vi "load_data.vi"(0 "datasource_pdf in":refnum<class "datasource_pdf.lvclass">, 11 "error in (no error)":errorcluster) -> (4 "datasource_pdf out":refnum<class "datasource_pdf.lvclass">, 6 "document":refnum<class "data_document.lvclass">[](array[class]), 15 "error out":errorcluster)   [LabVIEW 2020, in "datasource_pdf.lvclass"]
uses:
  datasource_pdf.lvclass
  data/data_document/data_document.lvclass
  datasource_pdf.lvclass/datasource_pdf.ctl
  models/message_image/message_image.lvclass
  D:/Personal/LabVIEW LLMs/src/models/abstract_message_base/abstract_message_base.lvclass
  models/message_image/create_image_message.vi
  models/message_text/get_text_message_value.vi
  utilities/pdf_utility/pdf_utility.lvlib
  models/abstract_llm_chatcompletion/abstract_llm_chatcompletion.lvclass
  models/message_text/message_text.lvclass
panel:
  out "pdf_path":string="  "
  # "Reading context from PDF using LLM"
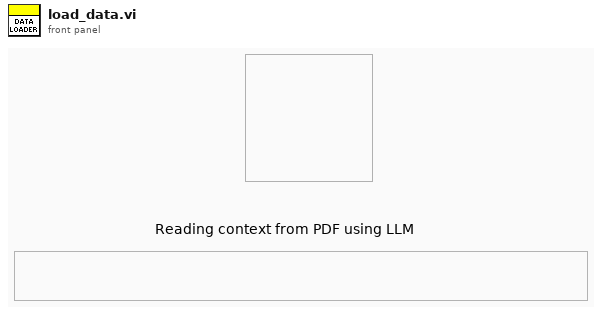
[diagram p1: front panel]
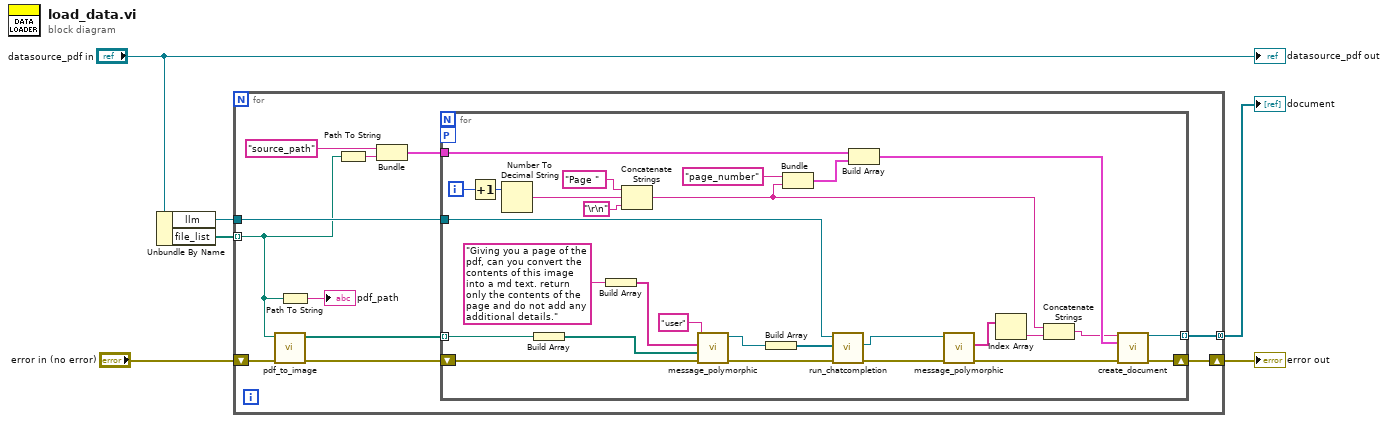
[diagram p0: block diagram]
diagram:
  n1 = Unbundle By Name("datasource_pdf in") -> ("llm"=w2:refnum<class "abstract_llm_base.lvclass">, "file_list"=w3:path[])
  n2 = for {
    shift-right: [w16] -> w4
    shift-left: "error in (no error)" -> [w17]
    tunnel: w3 -> [w7] mode=indexing
    tunnel: w2 -> [w12]
    tunnel: [w9] -> w1 mode=concatenating
    n3 = call "pdf_to_image.vi"("error in (no error)"=w17, "PDF File Path"=w7) -> ("error out"=w13:errorcluster, "Generated Images"=w11:path[])  [unwired: 8 in]
    n4 = Path To String(path=w7) -> (string=→"pdf_path":string)
    n5 = Path To String(path=w7) -> (string=w14:string)
    n6 = Bundle("source_path", w14) -> (w10:cluster{string, string})  [unwired: 1 in]
    n7 = for {
      tunnel: w12 -> [w42]
      shift-right: [w45] -> w16
      shift-left: w13 -> [w44]
      tunnel: w11 -> [w38] mode=indexing
      tunnel: w10 -> [w25]
      tunnel: [w20] -> w9 mode=indexing
      workers-P: _ -> [_]
      i -> [w28]
      n8 = Increment(x=w28) -> (x+1=w19:i32)
      n9 = Number To Decimal String(number=w19) -> (decimal integer string=w27:string)  [unwired: 1 in]
      n10 = Build Array(w38) -> (w37:path[])
      n11 = Build Array("Giving you a page of the pdf, can you convert the contents of this image into a md text. return only the contents of the page and do not add any additional details." ("text")) -> (w39:string[])
      n12 = Concatenate Strings("Page ", w27, "\r\n") -> (w21:string)
      n13 = call-poly "message_polymorphic.vi"("error in (no error)"=w44, "images"=w37, "text"=w39, "role"="user") -> ("error out"=w43:errorcluster, "message_text out"=w36:refnum<class "message_image.lvclass">)  [unwired: 6 in]
      n14 = Build Array(w36) -> (w35:refnum<class "message_image.lvclass">[])
      n15 = Bundle("page_number", w21) -> (w24:cluster{string, string})  [unwired: 1 in]
      n16 = call "run_chatcompletion.vi"("error in (no error)"=w43, "Messages"=w35, "abstract_llm_chatcompletion in"=w42) -> ("error out"=w33:errorcluster, "Response"=w31:refnum<class "abstract_message_base.lvclass">)  [unwired: 6 in, 1 out]
      n17 = Build Array(w25, w24) -> (w23:cluster{string, string}[])
      n18 = call-poly "message_polymorphic.vi"("error in"=w33, "abstract_message_base.lvclass"=w31) -> ("error out"=w32:errorcluster, "content"=w34:string[])  [unwired: 7 in, 1 out]
      n19 = Index Array(array=w34) -> (element=w30:string)  [unwired: 1 in]
      n20 = Concatenate Strings(w21, w30) -> (w22:string)
      n21 = call "create_document.vi"("text"=w22, "metadatas"=w23, "error in (no error)"=w32) -> ("data_document out"=w20:refnum<class "data_document.lvclass">, "error out"=w45:errorcluster)  [unwired: 11 in]
    }
  }
  "error out" <- w4
  "document" <- w1
  "datasource_pdf out" <- "datasource_pdf in"
